vi "HIT.vi"(0 "System no.":i32=1 min=1 max=4 step=1, 2 "TableID":i32[](array[numeric]), 3 "Value":dbl[](array[numeric]), 5 "error in":errorcluster, 6 "Address":i32[](array[numeric])) -> (19 "error out":errorcluster)   [LabVIEW 2020]
doc: "Sets values of custom lookup tables for Human Interface Devices (HID). See controller user manual for details. Requires Build SPA command substring.vi to be present.\n\nC-867: HIT writes the lookup tables in volatile memory only (RAM). Use WPA to save the current lookup table content to non-volatile memory. See controller user manual for details. \n\nC-884, E-871, E-872, E-873: HIT writes the lookup tables in volatile memory only (RAM). Use WPA to save the current lookup table content to non-volatile memory. See controller user manual for details."
panel:
  # "Sets values of custom lookup tables for Human Interface Devices (HID). See controller \nUser Manual for details. Requires \"Build SPA command substring.vi\" to be present."
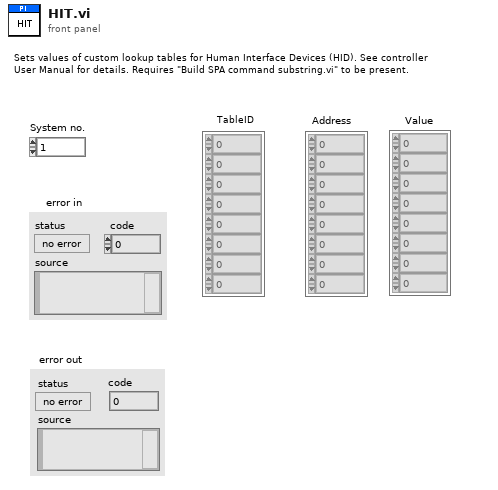
[diagram p1: front panel]
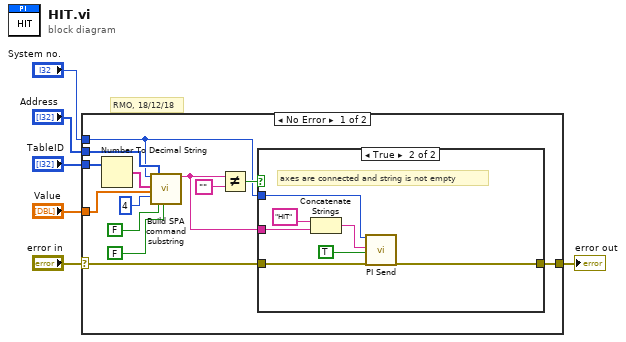
[diagram p0: block diagram]
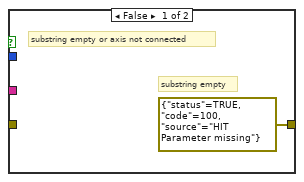
[diagram p2: hidden frame]
diagram:
  # "RMO, 18/12/18"
  n1 = case shown="No Error" "error in" {
    selector: "error in" -> [w7 w28]
    tunnel: [w19 w28] -> w6
    tunnel: "Value" -> [w16 _]
    tunnel: "System no." -> [w13 _]
    tunnel: "TableID" -> [w11 _]
    tunnel: "Address" -> [w15 _]
    frame No Error {
      n2 = Number To Decimal String(number=w11) -> (decimal integer string=w10:string[])  [unwired: 1 out]
      n3 = call "Build SPA command substring.vi"("System no."=w13, "Axes to set"=w10, "Parameter values"=w16, "No. of digits"=i16 4, "Parameter number"=w15, "Parameter no. format \n(Decimal: FALSE)"=FALSE ("Parameter no. format \n(Decimal: FALSE)"), "Parameter format \n(Num.: FALSE)"=FALSE ("Parameter format \n(Num.: FALSE)")) -> ("SPA command substring"=w17:string)  [unwired: 3 in, 9 out]
      n4 = Not Equal?(x=w17, y="") -> (x != y?=w14:bool)
      n5 = case shown="True" w14 {
        tunnel: w17 -> [_ w26]
        tunnel: [errorcluster {"status"=TRUE, "code"=100, "source"="HIT Parameter missing"} ("error out") w21] -> w19
        tunnel: w7 -> [_ w23]
        tunnel: w13 -> [_ w22]
        frame False {
          # "substring empty"
          # "substring empty or axis not connected"
        }
        frame True {
          # "axes are connected and string is not empty"
          n6 = Concatenate Strings("HIT", w26) -> (w24:string)
          n7 = call "PI Send.vi"("System no."=w22, "String to send"=w24, "Attach termination char.?"=TRUE ("Attach Linefeed?"), "error in"=w23) -> ("error out"=w21:errorcluster)  [unwired: 2 in, 13 out]
        }
      }
    }
    frame Error {
    }
  }
  "error out" <- w6
